vi "HexCenterFinder4Sides.vi"() -> ()   [LabVIEW 2019]
panel:
  out "appended array 3":dbl[](array[numeric])
  out "appended array 2":dbl[](array[numeric])
  out "appended array":dbl[](array[numeric])
  out "concatenated string":string
  out "S1":T1(plugin-control)
  out "InitialZ":dbl
  out "InitialY":dbl
  out "InitialX":dbl
  in  "HorizontalDistPCB":dbl=82.5
  in  "VerticalDistPCB":dbl=143.75
  in  "PCBEdges":path=path "C:/Users/TTUHEP/Documents/LabVIEW/Data/AssemblyIO_logs/BasePlateDefaultEdges.txt"
  in  "HorizontalDistSi":dbl=82.5
  in  "VerticalDistSi":dbl=143.75
  in  "SiEdges":path=path "C:/Users/TTUHEP/Documents/LabVIEW/Data/AssemblyIO_logs/BasePlateDefaultEdges.txt"
  out "S4":T1(plugin-control)
  out "S3":T1(plugin-control)
  out "S2":T1(plugin-control)
  in  "Component":enum16{"Baseplate", "Si", "PCB"}(ring)
  in  "VerticalDistBasePlate":dbl=143.75
  in  "HorizontalDistBasePlate":dbl=82.5
  in  "BasePlatePositions":path=path "C:/Users/TTUHEP/Documents/LabVIEW/Data/AssemblyIO_logs/BasePlateDefaultEdges.txt"
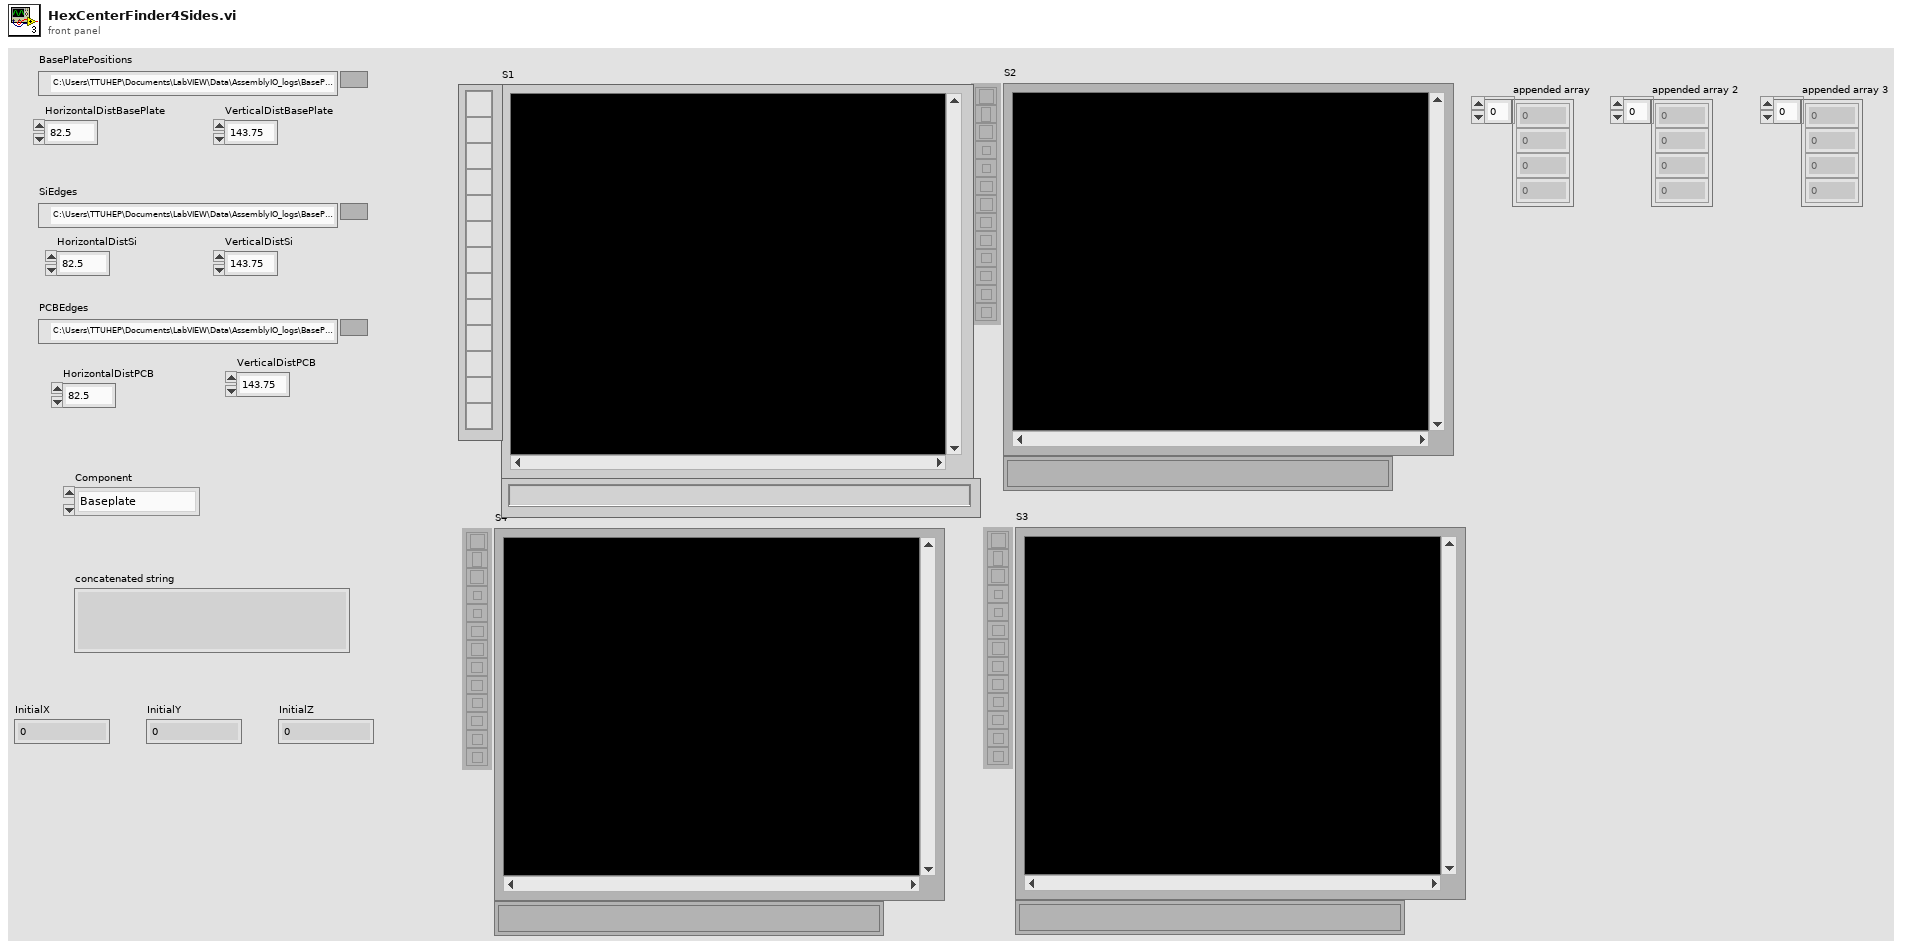
[diagram p1: front panel]
types:
  T1 = typedef "IMAQ Image.ctl" = refnum<image>
  T2 = typedef "IMAQ Line" = cluster{"Start X":i32, "Start Y":i32, "End X":i32, "End Y":i32}
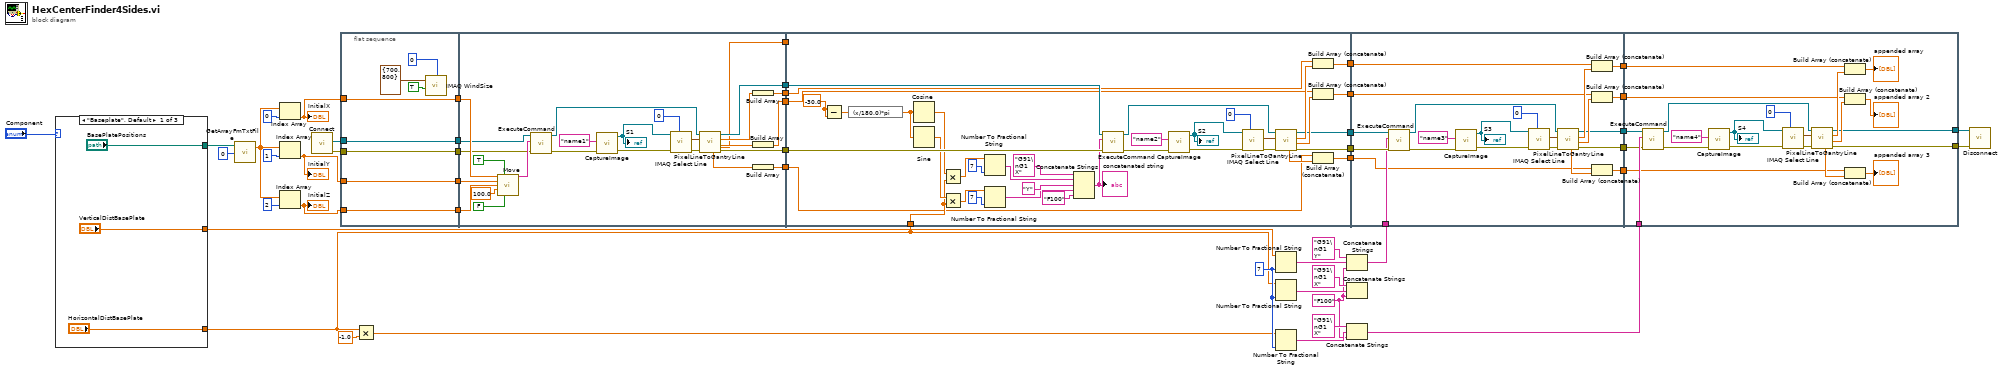
[diagram p0: block diagram]
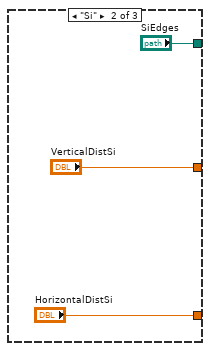
[diagram p2: hidden frame]
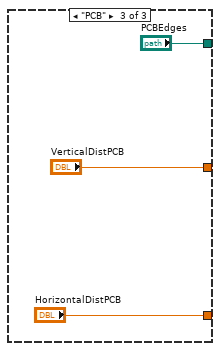
[diagram p3: hidden frame]
diagram:
  w20 = "F100" ("string")
  w30 = i16 7 ("precision (6)")
  n1 = case shown="\"Baseplate\", Default" "Component" {
    tunnel: ["BasePlatePositions" "SiEdges" "PCBEdges"] -> w43
    tunnel: ["VerticalDistBasePlate" "VerticalDistSi" "VerticalDistPCB"] -> w11
    tunnel: ["HorizontalDistBasePlate" "HorizontalDistSi" "HorizontalDistPCB"] -> w10
    frame "Baseplate", Default {
    }
    frame "Si" {
    }
    frame "PCB" {
    }
  }
  n2 = call "GetArrayFmTxtFile.vi"("LineNo."=0, "TextFile"=w43) -> ("Array"=w45:dbl[])  [unwired: 1 in, 1 out]
  n3 = Index Array(array=w45, index=0) -> (element=w42:dbl)
  "InitialX" <- w42
  n4 = Index Array(array=w45, index=1) -> (element=w14:dbl)
  "InitialY" <- w14
  n5 = Index Array(array=w45, index=2) -> (element=w13:dbl)
  "InitialZ" <- w13
  n6 = call "Connect.vi"() -> ("error out"=w41:errorcluster, "controller"=w40:refnum<k24>)  [unwired: 10 in]
  n7 = flat-sequence {
    tunnel: w40 -> [w62]
    tunnel: w41 -> [w63]
    tunnel: w13 -> [w64]
    tunnel: w14 -> [w65]
    tunnel: w42 -> [w66]
    tunnel: [w66] -> w19
    tunnel: [w65] -> w18
    tunnel: [w64] -> w17
    tunnel: [w63] -> w16
    tunnel: [w62] -> w15
    tunnel: [w77] -> w35
    tunnel: [w74] -> w34
    tunnel: w19 -> [w90]
    tunnel: w18 -> [w88]
    tunnel: w17 -> [w87]
    tunnel: w16 -> [w85]
    tunnel: w15 -> [w84]
    tunnel: [w68] -> w12
    tunnel: [w70] -> w9
    tunnel: [w69] -> w8
    tunnel: [w67] -> w7
    tunnel: w35 -> [w127]
    tunnel: w34 -> [w128]
    tunnel: [w98] -> w33
    tunnel: [w100] -> w32
    tunnel: w12 -> [_]
    tunnel: w10 -> [w110]
    tunnel: w9 -> [w97]
    tunnel: w8 -> [w96]
    tunnel: w7 -> [w95]
    tunnel: [w92] -> w6
    tunnel: [w94] -> w4
    tunnel: [w93] -> w3
    tunnel: w33 -> [w148]
    tunnel: w32 -> [w147]
    tunnel: w31 -> [w146]
    tunnel: [w138] -> w24
    tunnel: [w136] -> w23
    tunnel: w6 -> [w135]
    tunnel: [w129] -> w5
    tunnel: w4 -> [w134]
    tunnel: w3 -> [w133]
    tunnel: [w132] -> w2
    tunnel: [w131] -> w1
    tunnel: w25 -> [w170]
    tunnel: w24 -> [w169]
    tunnel: w23 -> [w168]
    tunnel: [w160] -> w22
    tunnel: [w157] -> w21
    tunnel: w5 -> [w159]
    tunnel: w2 -> [w156]
    tunnel: w1 -> [w155]
    frame #0 {
      n8 = call "IMAQ WindSize"("Scrollbars? (N)"=TRUE, "Width & Height"=cluster{"Width":i32, "Height":i32} {"Width"=700, "Height"=800}, "Window Number"=0) -> ()  [unwired: 3 in, 3 out]
    }
    frame #1 {
      n9 = call "Move.vi"("X"=w90, "Absolute"=TRUE, "Y"=w88, "Z"=w87, "SpeedXY (mm/s)"=100.0, "Move Z first"=FALSE) -> ("Position Gcode"=w91:string)  [unwired: 9 in]
      n10 = call "ExecuteCommand.vi"("error in (no error)"=w85, "Command Code"=w91, "controller in"=w84) -> ("error out"=w83:errorcluster, "controller out"=w78:refnum<k24>)  [unwired: 6 in, 1 out]
      n11 = call "CaptureImage.vi"("ImageName"="name1", "error in (no error)"=w83) -> ("Image"=w71:T1, "error out"=w79:errorcluster)  [unwired: 5 in]
      "S1" <- w71
      n12 = call "IMAQ Select Line"("Window Number (0...15)"=0, "error in (no error)"=w79, "Image In"=w71) -> ("error out"=w75:errorcluster, "Line"=w76:T2)  [unwired: 5 in, 2 out]
      n13 = call "PixelLineToGantryLine.vi"("error in"=w75, "cluster"=w76, "Controller In"=w78) -> ("error out"=w74:errorcluster, "intercept"=w72:dbl, "slope"=w73:dbl, "controller out"=w77:refnum<k24>, "Angle(degree)"=w68:dbl)  [unwired: 4 in]
      n14 = Build Array(w73) -> (w70:dbl[])
      n15 = Build Array(w72) -> (w69:dbl[])
      n16 = Build Array(w68) -> (w67:dbl[])
    }
    frame #2 {
      w109 = -30.0
      n17 = Subtract(x=w109, y=w109) -> (x-y=w111:dbl)
      n18 = expression code="(x/180.0)*pi"(w111) -> (w119:dbl)
      n19 = Cosine(x=w119) -> (cos(x)=w124:dbl)
      n20 = Sine(x=w119) -> (sin(x)=w118:dbl)
      n21 = Multiply(x=w124, y=w110) -> (x*y=w122:dbl)
      n22 = Multiply(x=w118, y=w110) -> (x*y=w120:dbl)
      n23 = Number To Fractional String(number=w122, precision (6)=i16 7) -> (F-format string=w116:string)  [unwired: 2 in]
      n24 = Number To Fractional String(number=w120, precision (6)=i16 7) -> (F-format string=w114:string)  [unwired: 2 in]
      n25 = Concatenate Strings("G91\nG1 X" ("string"), w116, "Y" ("string"), w114, "F100" ("string")) -> (w112:string)
      "concatenated string" <- w112
      n26 = call "ExecuteCommand.vi"("error in (no error)"=w128, "Command Code"=w112, "controller in"=w127) -> ("error out"=w125:errorcluster, "controller out"=w102:refnum<k24>)  [unwired: 6 in, 1 out]
      n27 = call "CaptureImage.vi"("ImageName"="name2", "error in (no error)"=w125) -> ("Image"=w99:T1, "error out"=w101:errorcluster)  [unwired: 5 in]
      "S2" <- w99
      n28 = call "IMAQ Select Line"("Window Number (0...15)"=0, "error in (no error)"=w101, "Image In"=w99) -> ("error out"=w106:errorcluster, "Line"=w107:T2)  [unwired: 5 in, 2 out]
      n29 = call "PixelLineToGantryLine.vi"("error in"=w106, "cluster"=w107, "Controller In"=w102) -> ("error out"=w100:errorcluster, "intercept"=w104:dbl, "slope"=w105:dbl, "controller out"=w98:refnum<k24>, "Angle(degree)"=w103:dbl)  [unwired: 4 in]
      n30 = Build Array (concatenate)(w97, w105) -> (w94:dbl[])
      n31 = Build Array (concatenate)(w96, w104) -> (w93:dbl[])
      n32 = Build Array (concatenate)(w95, w103) -> (w92:dbl[])
    }
    frame #3 {
      n33 = call "ExecuteCommand.vi"("error in (no error)"=w147, "Command Code"=w146, "controller in"=w148) -> ("error out"=w149:errorcluster, "controller out"=w137:refnum<k24>)  [unwired: 6 in, 1 out]
      n34 = call "CaptureImage.vi"("ImageName"="name3", "error in (no error)"=w149) -> ("Image"=w130:T1, "error out"=w139:errorcluster)  [unwired: 5 in]
      "S3" <- w130
      n35 = call "IMAQ Select Line"("Window Number (0...15)"=0, "error in (no error)"=w139, "Image In"=w130) -> ("error out"=w143:errorcluster, "Line"=w144:T2)  [unwired: 5 in, 2 out]
      n36 = call "PixelLineToGantryLine.vi"("error in"=w143, "cluster"=w144, "Controller In"=w137) -> ("error out"=w138:errorcluster, "intercept"=w141:dbl, "slope"=w142:dbl, "controller out"=w136:refnum<k24>, "Angle(degree)"=w140:dbl)  [unwired: 4 in]
      n37 = Build Array (concatenate)(w134, w142) -> (w132:dbl[])
      n38 = Build Array (concatenate)(w133, w141) -> (w131:dbl[])
      n39 = Build Array (concatenate)(w135, w140) -> (w129:dbl[])
    }
    frame #4 {
      n40 = call "ExecuteCommand.vi"("error in (no error)"=w169, "Command Code"=w170, "controller in"=w168) -> ("error out"=w171:errorcluster, "controller out"=w158:refnum<k24>)  [unwired: 6 in, 1 out]
      n41 = call "CaptureImage.vi"("ImageName"="name4", "error in (no error)"=w171) -> ("Image"=w151:T1, "error out"=w161:errorcluster)  [unwired: 5 in]
      "S4" <- w151
      n42 = call "IMAQ Select Line"("Window Number (0...15)"=0, "error in (no error)"=w161, "Image In"=w151) -> ("error out"=w165:errorcluster, "Line"=w166:T2)  [unwired: 5 in, 2 out]
      n43 = call "PixelLineToGantryLine.vi"("error in"=w165, "cluster"=w166, "Controller In"=w158) -> ("error out"=w160:errorcluster, "intercept"=w163:dbl, "slope"=w164:dbl, "controller out"=w157:refnum<k24>, "Angle(degree)"=w162:dbl)  [unwired: 4 in]
      n44 = Build Array (concatenate)(w156, w164) -> (→"appended array":dbl[])
      n45 = Build Array (concatenate)(w155, w163) -> (→"appended array 2":dbl[])
      n46 = Build Array (concatenate)(w159, w162) -> (→"appended array 3":dbl[])
    }
  }
  n47 = Multiply(x=w10, y=-1.0) -> (x*y=w26:dbl)
  n48 = Number To Fractional String(number=w11, precision (6)=w30) -> (F-format string=w36:string)  [unwired: 2 in]
  n49 = Number To Fractional String(number=w10, precision (6)=w30) -> (F-format string=w38:string)  [unwired: 2 in]
  n50 = Number To Fractional String(number=w26, precision (6)=w30) -> (F-format string=w28:string)  [unwired: 2 in]
  n51 = Concatenate Strings("G91\nG1 Y" ("string"), w36, w20) -> (w31:string)
  n52 = Concatenate Strings("G91\nG1 X" ("string"), w38, w20) -> ()  [unwired: 1 out]
  n53 = Concatenate Strings("G91\nG1 X" ("string"), w28, w20) -> (w25:string)
  n54 = call "Disconnect.vi"("error in (no error)"=w22, "controller"=w21) -> ()  [unwired: 9 in, 1 out]
